vi "optionsAcq_channel_attenuatorAuto.vi"(8 "error in (no error)":errorcluster, 9 "readWrite":enum16{"read", "write"}(ring), 10 "attenuator auto":bool, 11 "OSAchannel in":refnum<class "OSAchannel.lvclass">) -> (0 "error out":errorcluster, 1 "FTSLib status":i32, 2 "auto read":bool, 3 "OSAchannel out":refnum<class "OSAchannel.lvclass">)   [LabVIEW 2010, in "OSAchannel.lvclass"]
uses:
  OSAchannel.lvclass
  OSAchannel.lvclass/OSAchannel.ctl
  _dll/LVLib/FTSLib.lvlib
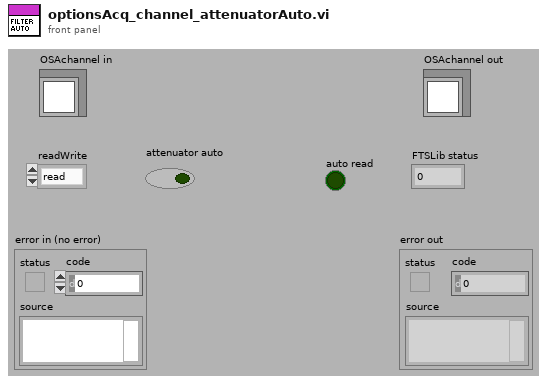
[diagram p1: front panel]
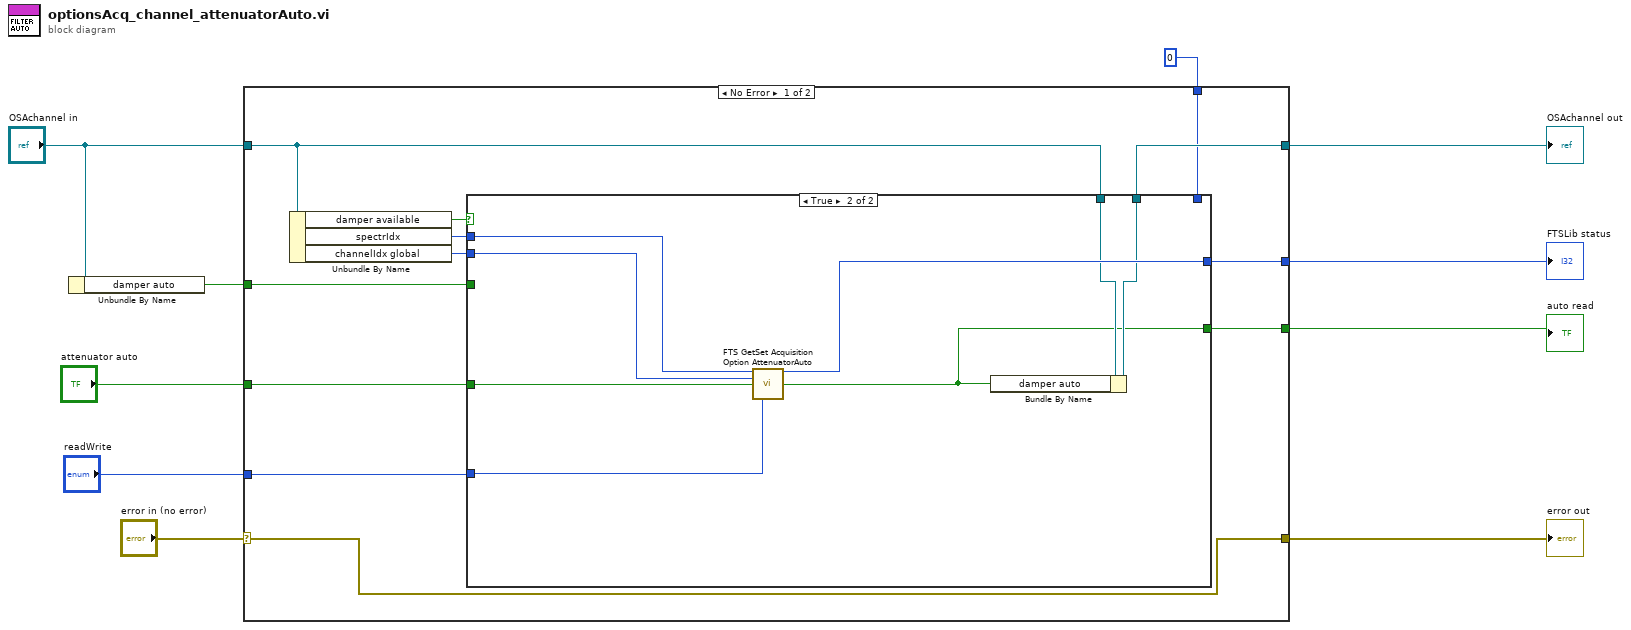
[diagram p0: block diagram]
diagram:
  n1 = Unbundle By Name("OSAchannel in") -> ("damper auto"=w2:bool)
  n2 = case shown="No Error" "error in (no error)" {
    selector: "error in (no error)" -> [w13 w37]
    tunnel: [w13 w37] -> w9
    tunnel: [w14 w36] -> w8
    tunnel: "OSAchannel in" -> [w15 w36]
    tunnel: "readWrite" -> [w21 _]
    tunnel: "attenuator auto" -> [w18 _]
    tunnel: [w17 w34] -> w5
    tunnel: [w16 w35] -> w4
    tunnel: w2 -> [w11 w35]
    tunnel: 0 ("FTSLib status") -> [w12 w34]
    frame No Error {
      n3 = Unbundle By Name(w15) -> ("damper available"=w22:bool, "spectrIdx"=w20:u16, "channelIdx global"=w19:u16)
      n4 = case shown="True" w22 {
        tunnel: w21 -> [_ w33]
        tunnel: w20 -> [_ w32]
        tunnel: w19 -> [_ w31]
        tunnel: w18 -> [_ w30]
        tunnel: [w24 w29] -> w17
        tunnel: [w23 w26] -> w16
        tunnel: w15 -> [w25 w28]
        tunnel: [w25 w27] -> w14
        tunnel: w12 -> [w24 _]
        tunnel: w11 -> [w23 _]
        frame False {
        }
        frame True {
          n5 = call "FTS GetSet Acquisition Option AttenuatorAuto.vi"("spectrIdx"=w32, "channel"=w31, "attenuator auto"=w30, "readWrite"=w33) -> ("FTSLib status"=w29:i32, "auto read"=w26:bool)  [unwired: 10 in]
          n6 = Bundle By Name(cluster=w28, "damper auto"=w26) -> (w27:refnum<class "OSAchannel.lvclass">)
        }
      }
    }
    frame Error {
    }
  }
  "error out" <- w9
  "OSAchannel out" <- w8
  "FTSLib status" <- w5
  "auto read" <- w4
